vi "input.vi"(9 "Z":dbl, 10 "Y":dbl, 11 "X":dbl) -> (3 "yo":dbl[](array[numeric]))   [LabVIEW 2015]
uses:
  <vilib>/imath/engines/lvmath2/RunTimeEngine/ArithmeticOperatorToken/NIMS_ArithmeticOperator_multmx(M,CV)-internal.vi
  <instcachedir>/0/NIMS_ArithmeticOperator_multmx(M,CV)-internal_4015640DB52447B392A036248F93EE7C.lvgen/NIMS_ArithmeticOperator_multmx(M,CV)-internal_4015640DB52447B392A036248F93EE7C_001.vi
  <vilib>/imathl/engines/lvmath/Functions/Error Handling/Create Error.vi
  <vilib>/imath/engines/lvmath2/RunTimeEngine/NodeEndStatement/NIMS_NodeEndStatement_Output.vi
  <instcachedir>/0/NIMS_NodeEndStatement_Output_53EC0D466D134D7ABD903AC30B43404B.lvgen/NIMS_NodeEndStatement_Output_53EC0D466D134D7ABD903AC30B43404B_005.vi
  <vilib>/imath/engines/lvmath2/RunTimeEngine/ErrorHandling/NIMS_Finalize Error.vi
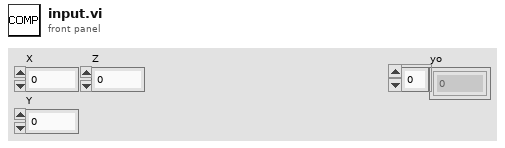
[diagram p1: front panel]
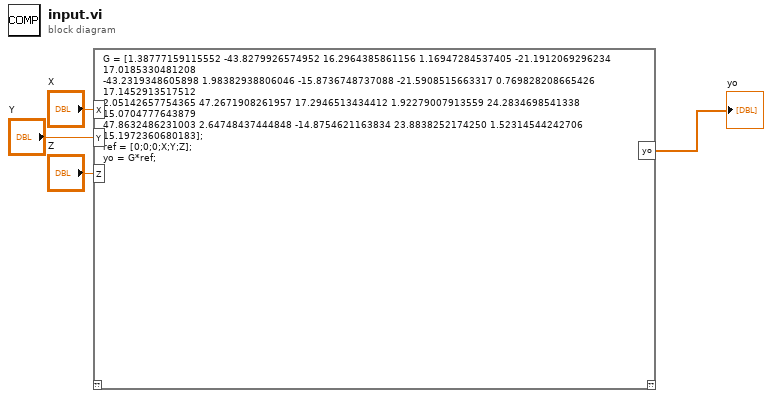
[diagram p0: block diagram]
diagram:
  n1 = mathscript code="G = [1.38777159115552\t-43.8279926574952\t16.2964385861156\t1.16947284537405\t-21.1912069296234\t17.0185330481208\n-43.2319348605898\t1.98382938806046\t-15.8736748737088\t-21.5908515663317\t0.769828208665426\t17.1452913517512\n2.05142657754365\t47.2671908261957\t17.2946513434412\t1.92279007913559\t24.2834698541338\t15.0704777643879\n47.8632486231003\t2.64748437444848\t-14.8754621163834\t23.8838252174250\t1.52314544242706\t15.1972360680183];\nref = [0;0;0;X;Y;Z];\nyo = G*ref;"("X"="X", "Y"="Y", "Z"="Z") -> ("yo"=→"yo":dbl[])  [unwired: 1 in, 1 out]
